vi "set position windmill.vi"(6 "Args":string[](array[string]), 7 "device_reference":i32, 8 "error in (no error)":errorcluster, 9 "String":string, 10 "Settings":T1={"device_name"="", "pitch"={"Value"=0.0, "Min"=0.0, "Max"=0.0, "StepSize"=0.0, "Tolerance"=0.0, "ValueActual"=0.0}, "position"={"Value"=0.0, "Min"=0.0, "Max"=0.0, "StepSize"=0.0, "Tolerance"=0.0, "ValueActual"=0.0}, "lowspeed"={"Value"=0.0, "Min"=0.0, "Max"=0.0, "StepSize"=0.0, "Tolerance"=0.0, "ValueActual"=0.0}, "highspeed"={"Value"=0.0, "Min"=0.0, "Max"=0.0, "StepSize"=0.0, "Tolerance"=0.0, "ValueActual"=0.0}, "motor_status"=enum."off", "InitDelay"={"Value"=0.0, "Min"=0.0, "Max"=0.0, "StepSize"=0.0, "Tolerance"=0.0, "ValueActual"=0.0}, "stepsequence"=[], "step"=enum."off", "AutoStep"=enum."off", "MinMonMaxCounts"={"Value"=1000.0, "Min"=0.0, "Max"=0.0, "StepSize"=0.0, "Tolerance"=0.0, "ValueActual"=0.0}, "MinMonMeanCountsRaw"={"Value"=1000.0, "Min"=0.0, "Max"=0.0, "StepSize"=0.0, "Tolerance"=0.0, "ValueActual"=0.0}, "AutoStepTimeout"={"Value"=30000.0, "Min"=0.0, "Max"=0.0, "StepSize"=0.0, "Tolerance"=0.0, "ValueActual"=0.0}}, 11 "WindmillDevice in":refnum<class "WindmillDevice.lvclass">) -> (0 "error out":errorcluster, 2 "new commands":string, 3 "WindmillDevice out":refnum<class "WindmillDevice.lvclass">)   [LabVIEW 2020, in "WindmillDevice.lvclass"]
uses:
  WindmillDevice.lvclass
  settingsArcus_TypDef.ctl
  shared/numericVariable_TypeDef.ctl
  WindmillDevice.lvclass/WindmillDevice.ctl
  shared/CompressAndUpdate(Poly)/CompressAndUpdate(Numeric).vi
  BaseDriver/BaseDriver.lvclass
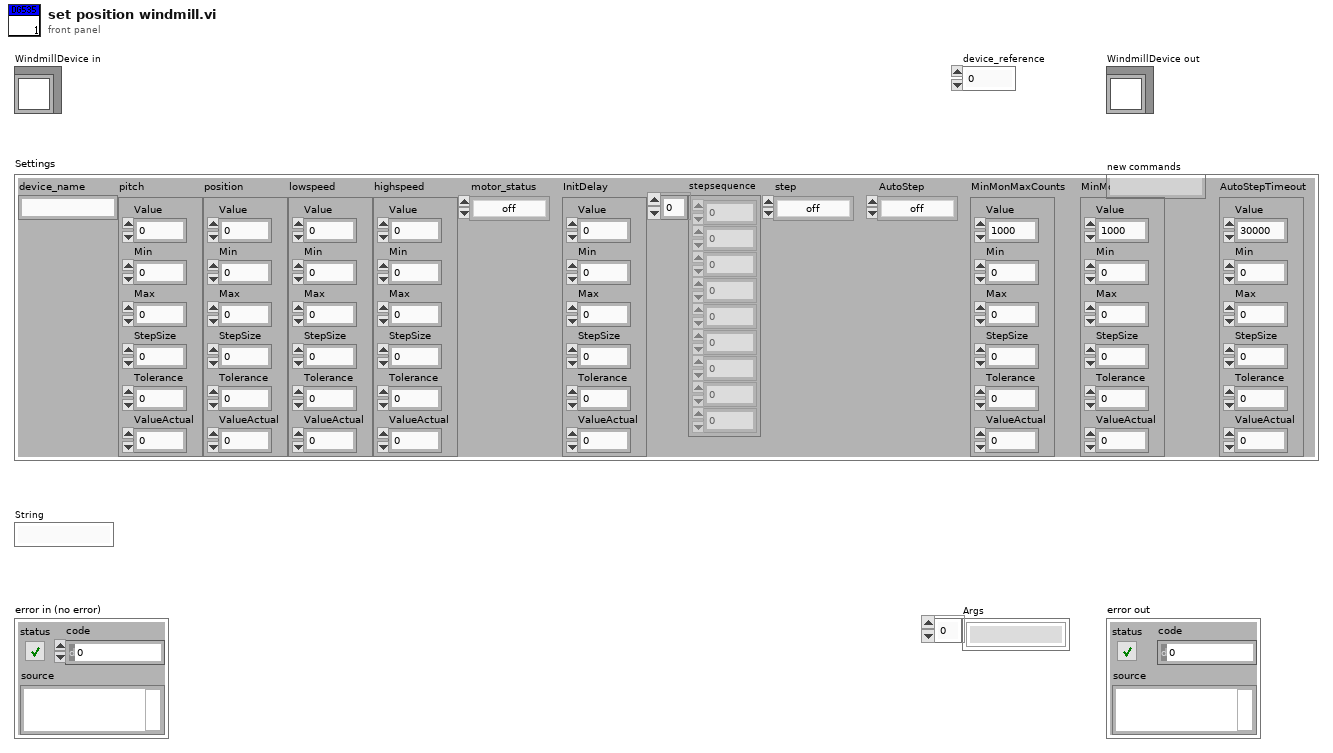
[diagram p1: front panel]
types:
  T1 = typedef "WindmillDevice.lvclass/settingsArcus_TypDef.ctl" = cluster{"device_name":string, "pitch":T2, "position":T2, "lowspeed":T2, "highspeed":T2, "motor_status":enum16{"off", "on"}, "InitDelay":T2, "stepsequence":dbl[], "step":enum16{"off", "on"}, "AutoStep":enum16{"off", "on"}, "MinMonMaxCounts":T2, "MinMonMeanCountsRaw":T2, "AutoStepTimeout":T2}
  T2 = typedef "BaseDriver.lvclass/numericVariable_TypeDef.ctl" = cluster{"Value":dbl, "Min":dbl, "Max":dbl, "StepSize":dbl, "Tolerance":dbl, "ValueActual":dbl}
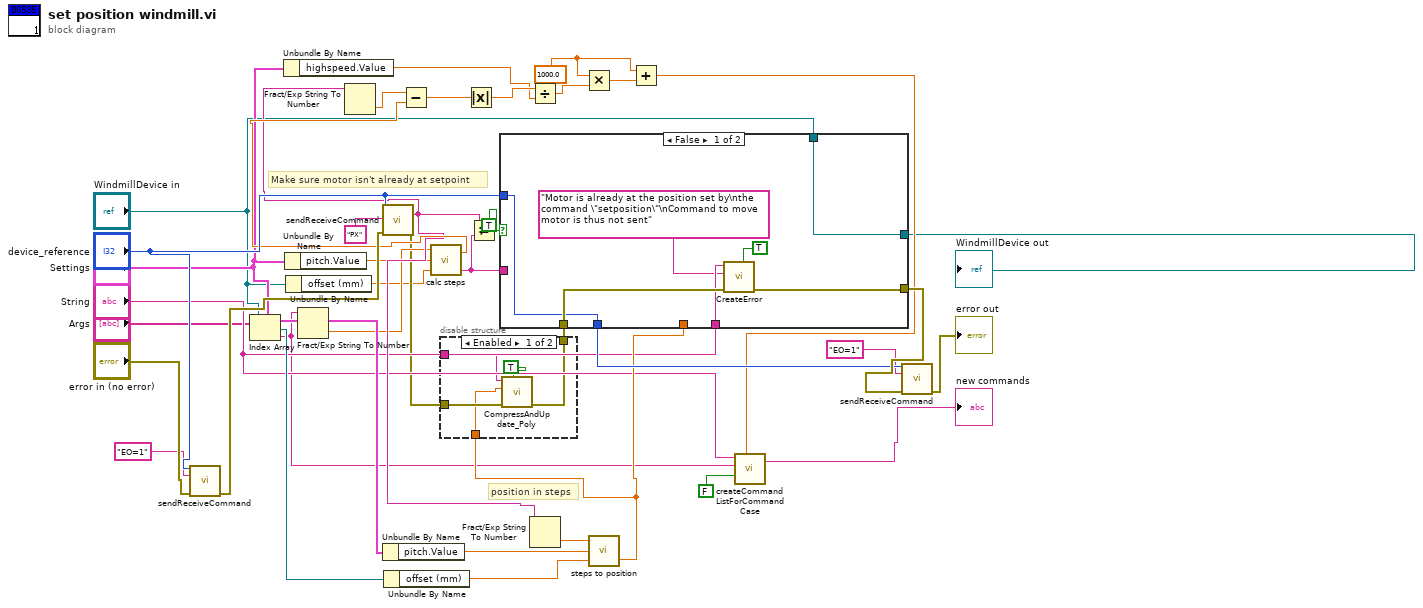
[diagram p0: block diagram]
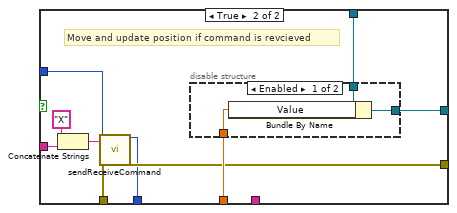
[diagram p3: hidden frame]
diagram:
  w30 = 1000.0 ("x")
  # "position in steps"
  # "Make sure motor isn't already at setpoint"
  n1 = call "sendReceiveCommand.vi"("reference (in)"="device_reference", "write_string"="EO=1", "error in (no error)"="error in (no error)") -> ("error out"=w34:errorcluster)  [unwired: 10 in, 2 out]
  n2 = Index Array(array="Args") -> (element=w6:string)  [unwired: 1 in]
  n3 = Unbundle By Name("Settings") -> ("highspeed.Value"=w25:dbl)
  n4 = Unbundle By Name("Settings") -> ("pitch.Value"=w8:dbl)
  n5 = Unbundle By Name("WindmillDevice in") -> ("offset (mm)"=w9:dbl)
  n6 = Fract/Exp String To Number(string=w6) -> (number=w14:dbl)  [unwired: 3 in, 1 out]
  n7 = call "sendReceiveCommand.vi"("reference (in)"="device_reference", "write_string"="PX", "error in (no error)"=w34) -> ("read_string"=w21:string, "error out"=w10:errorcluster)  [unwired: 10 in, 1 out]
  n8 = Fract/Exp String To Number(string=w21) -> (number=w22:dbl)  [unwired: 3 in, 1 out]
  n9 = Unbundle By Name("Settings") -> ("pitch.Value"=w16:dbl)
  n10 = Unbundle By Name("WindmillDevice in") -> ("offset (mm)"=w17:dbl)
  n11 = call "calc steps.vi"("Offset (mm)"=w9, "Pitch"=w8, "Position to set (mm)"=w14) -> ("# counts"=w1:string, "pos to set (steps)"=w23:dbl)
  n12 = Subtract(x=w22, y=w23) -> (x-y=w24:dbl)
  n13 = Absolute Value(x=w24) -> (abs(x)=w28:dbl)
  n14 = Not Equal?(x=w21, y=w1) -> ()  [unwired: 1 out]
  n15 = Divide(x=w28, y=w25) -> (x/y=w26:dbl)
  n16 = Fract/Exp String To Number(string=w21) -> (number=w15:dbl)  [unwired: 3 in, 1 out]
  n17 = Multiply(x=w30, y=w26) -> (x*y=w27:dbl)
  n18 = call "steps to position.vi"("Offset (mm)"=w17, "Pitch"=w16, "position (steps)"=w15) -> ("Position  (mm)"=w19:dbl)  [unwired: 1 in]
  n19 = disable-structure shown="Enabled" {
    disable-tunnel: w10 -> [w42 _]
    disable-tunnel: [w41 _] -> w11
    disable-tunnel: "String" -> [w40 _]
    disable-tunnel: w19 -> [w39 _]
    frame Enabled {
      n20 = call-poly "CompressAndUpdate_Poly.vi"("force CVT update (false)"=TRUE, "error in"=w42, "Numeric"=w39, "command or variable name"=w40) -> ("error out"=w41:errorcluster)  [unwired: 7 in]
    }
    frame Disabled {
    }
  }
  n21 = case shown="False" TRUE {
    tunnel: "device_reference" -> [w44 w58]
    tunnel: w1 -> [_ w57]
    tunnel: w11 -> [w49 w56]
    tunnel: "WindmillDevice in" -> [w50 w55]
    tunnel: w19 -> [_ w54]
    tunnel: [w48 w53] -> w37
    tunnel: [w50 w52] -> w3
    tunnel: "String" -> [w47 _]
    tunnel: [w44 w51] -> w36
    frame False {
      n22 = call "CreateError.vi"("Warning"=TRUE, "user error in"=w49, "error message (\"\")"="Motor is already at the position set by\nthe command \"setposition\"\nCommand to move motor is thus not sent" ("error message (\"\")"), "command"=w47) -> ("user error  out"=w48:errorcluster)  [unwired: 7 in]
    }
    frame True {
      # "Move and update position if command is revcieved"
      n23 = Concatenate Strings("X" ("raw_cmd"), w57) -> (w59:string)
      n24 = call "sendReceiveCommand.vi"("reference (in)"=w58, "write_string"=w59, "error in (no error)"=w56) -> ("reference (out)"=w51:i32, "error out"=w53:errorcluster)  [unwired: 10 in, 1 out]
      n25 = disable-structure shown="Enabled" {
        disable-tunnel: w55 -> [w63 w64]
        disable-tunnel: w54 -> [w62 _]
        disable-tunnel: [w61 w64] -> w52
        frame Enabled {
          n26 = Bundle By Name(cluster=w63, "Value"=w62) -> (w61:refnum<class "WindmillDevice.lvclass">)
        }
        frame Disabled {
        }
      }
    }
  }
  "WindmillDevice out" <- w3
  n27 = Add(x=w30, y=w27) -> (x+y=w29:dbl)
  n28 = call "createCommandListForCommandCase.vi"("timeout (optional)"=w29, "immediate Check (only once)"=FALSE, "setvalue"=w6, "command"="String") -> ("new commands"=→"new commands":string)  [unwired: 7 in]
  n29 = call "sendReceiveCommand.vi"("reference (in)"=w36, "write_string"="EO=1", "error in (no error)"=w37) -> ("error out"=→"error out":errorcluster)  [unwired: 10 in, 2 out]
